vi "update_biases.vi"(6 "Back Output":dbl[](array[numeric]), 9 "Delta":dbl[](array[numeric]), 10 "Learning Parameter":dbl, 11 "Biases":dbl[](array[numeric])) -> (3 "Updated Biases":dbl[](array[numeric]))   [LabVIEW 2018]
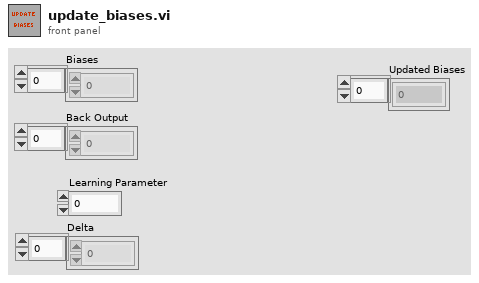
[diagram p1: front panel]
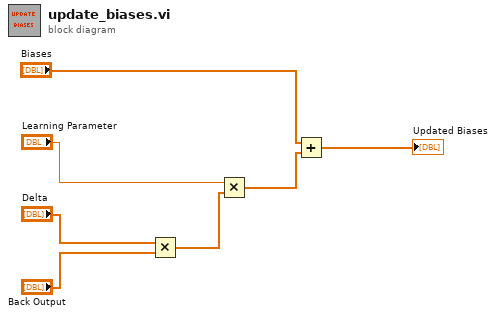
[diagram p0: block diagram]
diagram:
  n1 = Multiply(x="Delta", y="Back Output") -> (x*y=w4:dbl[])
  n2 = Multiply(x="Learning Parameter", y=w4) -> (x*y=w2:dbl[])
  n3 = Add(x="Biases", y=w2) -> (x+y=→"Updated Biases":dbl[])
